vi "Init Actor Core.vi"(8 "error in (no error)":errorcluster, 11 "Interactive Tree in":refnum<class "Interactive Tree.lvclass">) -> (0 "error out":errorcluster, 3 "Interactive Tree out":refnum<class "Interactive Tree.lvclass">)   [LabVIEW 2016]
uses:
  Interactive Tree.lvclass
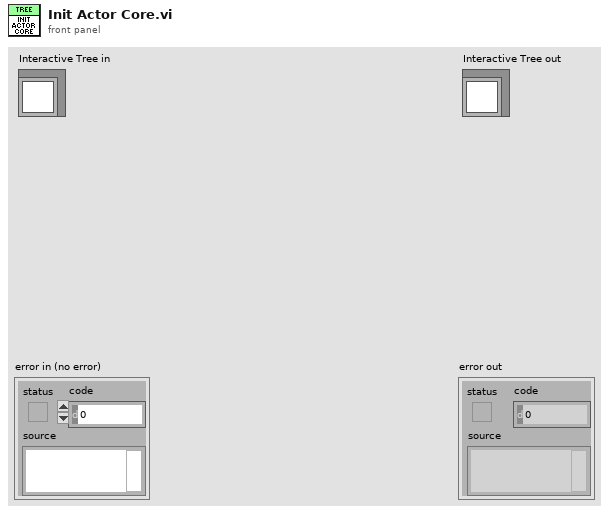
[diagram p1: front panel]
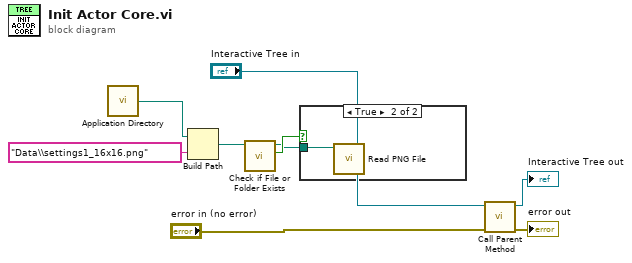
[diagram p0: block diagram]
diagram:
  n1 = call <vilib>:"Application Directory.vi"() -> ("Application Directory"=w3:path)
  n2 = Build Path(base path=w3, name or relative path="Data\\settings1_16x16.png") -> (appended path=w4:path)
  n3 = call <vilib>:"Check if File or Folder Exists.vi"("path"=w4) -> ("file or folder exists?"=w2:bool, "dup path"=w1:path)  [unwired: 8 in, 1 out]
  n4 = case shown="True" w2 {
    tunnel: w1 -> [_ w10]
    frame False {
    }
    frame True {
      n5 = call <vilib>:"Read PNG File.vi"("path to PNG file"=w10) -> ()  [unwired: 8 in, 3 out]
    }
  }
  n6 = call-parent "Call Parent Method"("error in (no error)"="error in (no error)", "Measure Object in"="Interactive Tree in") -> ("error out"=→"error out":errorcluster, "Measure Object out"=→"Interactive Tree out":refnum<class "Interactive Tree.lvclass">)  [unwired: 8 in]
